vi "UI_visual.vi"() -> ()   [LabVIEW 2017]
uses:
  <vilib>/Analysis/coordinate.llb/Euler Rotation Order.ctl
  <vilib>/Utility/miscctls.llb/LV3DPointTypeDef.ctl
  <vilib>/Analysis/baseanly.llb/Real A x B.vi
  <vilib>/Analysis/Matrix/Numeric/Conversions/Array To Matrix - RA.vi
  <vilib>/Analysis/Matrix/Numeric/Conversions/Array To Matrix - RA2.vi
  <vilib>/Analysis/Matrix/Numeric/Conversions/Matrix To Array - RM.vi
  <vilib>/picture/3D Picture Control/Object/Create Object (drawable).vi
  <vilib>/picture/3D Picture Control/Object/Create Object (name).vi
  <vilib>/picture/3D Picture Control/Object/Add Object (no reference).vi
  <vilib>/picture/3D Picture Control/Helpers/Set Clip Plane (no reference).vi
  <vilib>/picture/3D Picture Control/Helpers/Apply Texture (no reference).vi
  <vilib>/picture/3D Picture Control/NI_3D Picture Control.lvlib
  <vilib>/Analysis/NI_AALPro.lvlib
  <vilib>/Analysis/Matrix/NI_Matrix.lvlib
  <vilib>/Analysis/NI_AALBase.lvlib
panel:
  out "Euler_angles recebidos":dbl[](array[numeric])
  out "Euler Angles":dbl[](array[numeric])
  out "alt":dbl
  out "B-frame":cluster{"X":sgl, "Y":sgl, "Z":sgl}
  out "array":dbl[](array[numeric])
  in  "B-frame Translation 2":cluster{"X":sgl, "Y":sgl, "Z":sgl}
  in  "N-frame rot":dbl[](array[numeric])
  in  "N-frame Translation":cluster{"X":sgl, "Y":sgl, "Z":sgl}
  in  "B-frame Translation":cluster{"X":sgl, "Y":sgl, "Z":sgl}
  in  "Up Direction":T1={"X"=0.0, "Y"=0.0, "Z"=1.0}
  out "3D Picture Control":refnum<vi>(3d-picture)
  in  "error in (no error)":errorcluster
  in  "rotation order":T2 items=["X-Y-Z", "X-Z-Y", "Y-X-Z", "Y-Z-X", "Z-X-Y", "Z-Y-X", "X-Y-X", "X-Z-X", "Y-X-Y", "Y-Z-Y", "Z-X-Z", "Z-Y-Z"]
  in  "Rodar nesta VI":bool
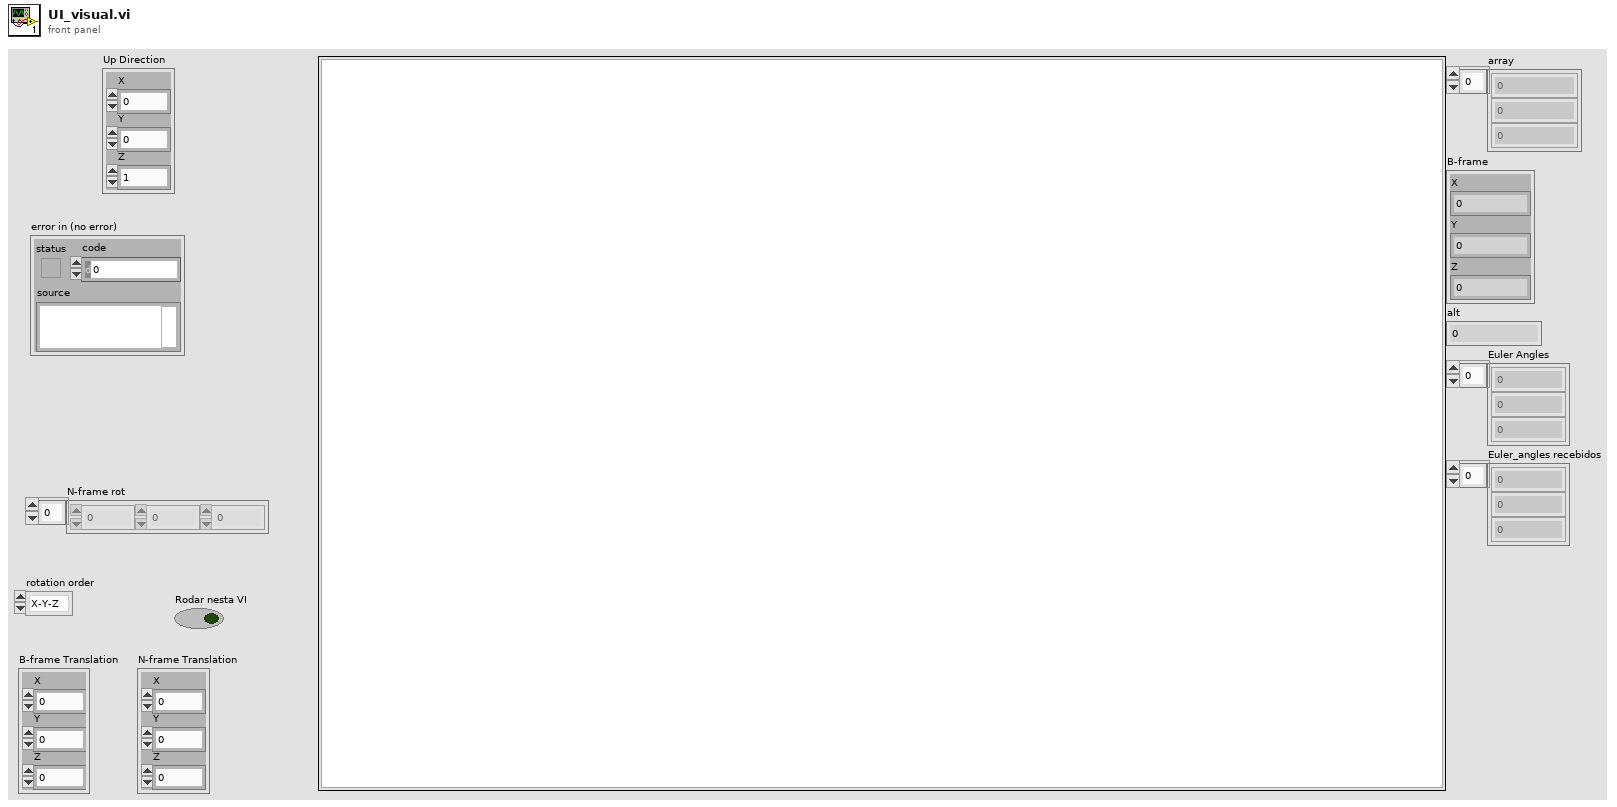
[diagram p1: front panel]
types:
  T1 = typedef "LV3DPointTypeDef.ctl" = cluster{"X":sgl, "Y":sgl, "Z":sgl}
  T2 = typedef "NI_AALPro.lvlib/Euler Rotation Order.ctl" = u16
  T3 = cluster{"Red":sgl, "Green":sgl, "Blue":sgl, "Alpha":sgl}
  T4 = enum16{"As a Decal", "With Modulation", "With Blending", "As a replacement"}
  T5 = enum16{"Inherit Value", "Points", "Wireframe", "Polygons"}
  T6 = typedef "NI_Matrix.lvlib/RealMatrix.ctl" = dbl[][]
  T7 = typedef "imagedata.ctl" = cluster{"image type":i32, "image depth":i32, "image":u8[], "mask":u8[], "colors":u32[], "Rectangle":cluster{"left":i16, "top":i16, "right":i16, "bottom":i16}}
  T8 = cluster{"element":dbl, "element":dbl, "element":dbl}
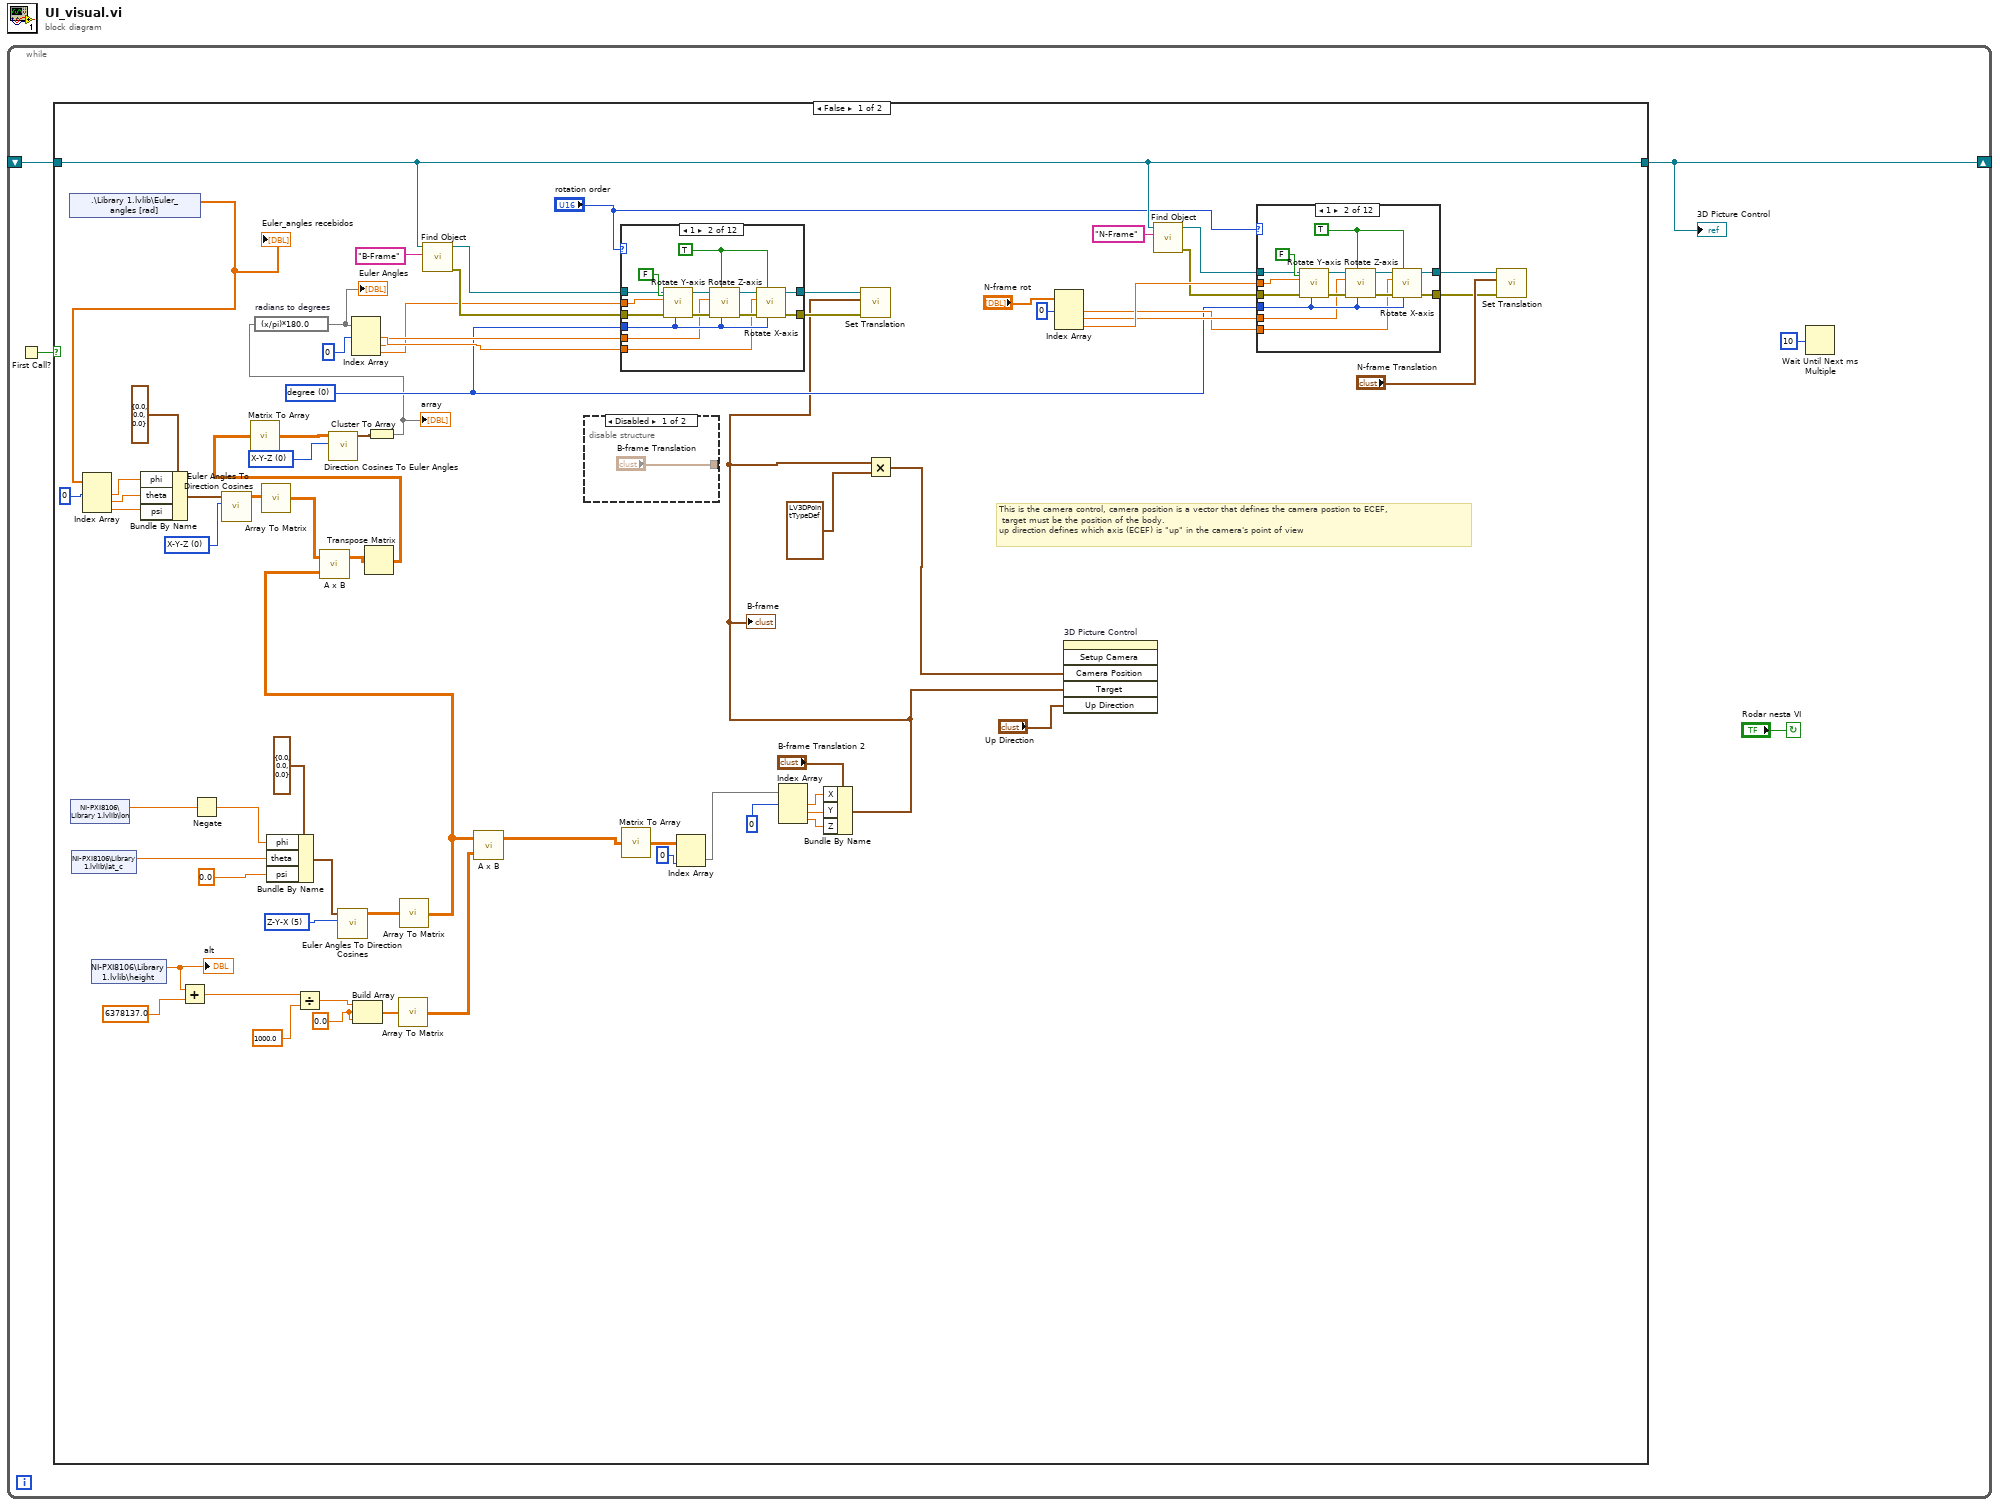
[diagram p0: block diagram]
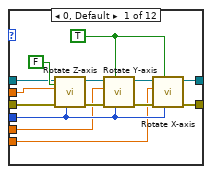
[diagram p3: hidden frame]
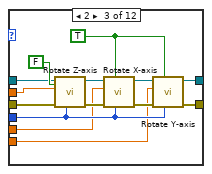
[diagram p4: hidden frame]
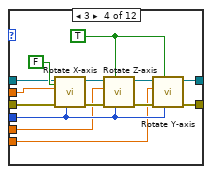
[diagram p5: hidden frame]
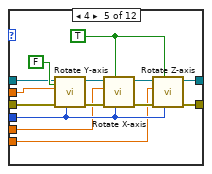
[diagram p6: hidden frame]
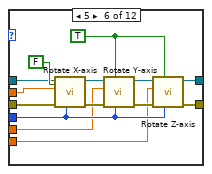
[diagram p7: hidden frame]
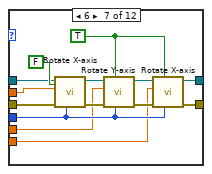
[diagram p8: hidden frame]
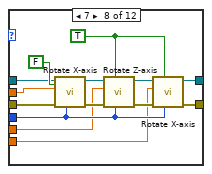
[diagram p9: hidden frame]
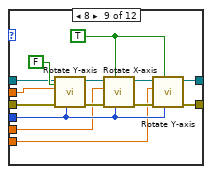
[diagram p10: hidden frame]
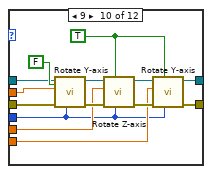
[diagram p11: hidden frame]
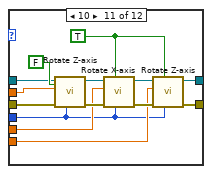
[diagram p12: hidden frame]
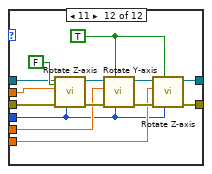
[diagram p13: hidden frame]
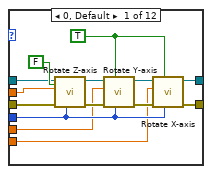
[diagram p14: hidden frame]
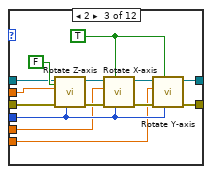
[diagram p15: hidden frame]
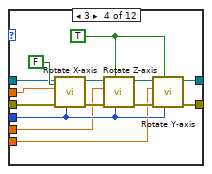
[diagram p16: hidden frame]
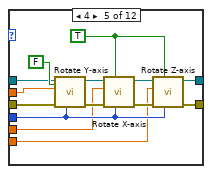
[diagram p17: hidden frame]
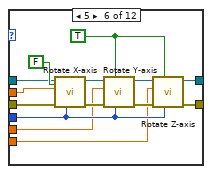
[diagram p18: hidden frame]
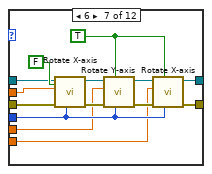
[diagram p19: hidden frame]
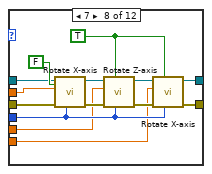
[diagram p20: hidden frame]
diagram:
  n1 = while {
    shift-right: [w2] -> _
    shift-left: _ -> [w3]
    stop <- "Rodar nesta VI" continue-if-true
    n2 = First Call?() -> (First Call?: T/F=w5:bool)
    n3 = case shown="False" w5 {
      tunnel: [w53 w425] -> w2
      tunnel: w3 -> [w53 _]
      frame False {
        w16 = T2 0 items=["X-Y-Z", "X-Z-Y", "Y-X-Z", "Y-Z-X", "Z-X-Y", "Z-Y-X", "X-Y-X", "X-Z-X", "Y-X-Y", "Y-Z-Y", "Z-X-Z", "Z-Y-Z"] ("rotation order")
        w27 = T2 0 items=["X-Y-Z", "X-Z-Y", "Y-X-Z", "Y-Z-X", "Z-X-Y", "Z-Y-X", "X-Y-X", "X-Z-X", "Y-X-Y", "Y-Z-Y", "Z-X-Z", "Z-Y-Z"] ("rotation order")
        w42 = 0.0 ("element")
        w50 = T2 5 items=["X-Y-Z", "X-Z-Y", "Y-X-Z", "Y-Z-X", "Z-X-Y", "Z-Y-X", "X-Y-X", "X-Z-X", "Y-X-Y", "Y-Z-Y", "Z-X-Z", "Z-Y-Z"] ("rotation order")
        w51 = u16 0 items=["degree", "radians"] ("angle unit")
        # "This is the camera control, camera position is a vector that defines the camera postion to ECEF,\n target must be the position of the body. \nup direction defines which axis (ECEF) is \"up\" in the camera's point of view"
        n4 = shared-variable ".\\Library 1.lvlib\\Euler_angles [rad]"() -> (w6:dbl[])  [unwired: 1 in, 1 out]
        "Euler_angles recebidos" <- w6
        n5 = shared-variable "NI-PXI8106\\Library 1.lvlib\\lon"() -> (w10:dbl)  [unwired: 1 in, 1 out]
        n6 = shared-variable "NI-PXI8106\\Library 1.lvlib\\lat_c"() -> (w11:dbl)  [unwired: 1 in, 1 out]
        n7 = Index Array(array=w6, index #1=0 ("index")) -> (element #1=w25:dbl, element #2=w24:dbl, element #3=w23:dbl)  [unwired: 2 in]
        n8 = shared-variable "NI-PXI8106\\Library 1.lvlib\\height"() -> (w46:dbl)  [unwired: 1 in, 1 out]
        "alt" <- w46
        n9 = Bundle By Name(cluster=cluster{"phi":dbl, "theta":dbl, "psi":dbl} {"phi"=0.0, "theta"=0.0, "psi"=0.0} ("Euler Angles"), "phi"=w25, "theta"=w24, "psi"=w23) -> (w28:cluster{"phi":dbl, "theta":dbl, "psi":dbl})
        n10 = Add(x=w46, y=6378137.0) -> (x+y=w44:dbl)
        n11 = Negate(x=w10) -> (-x=w9:dbl)
        n12 = call <vilib>:"Euler Angles To Direction Cosines.vi"("rotation order"=w27, "Euler Angles"=w28) -> ("Direction Cosines"=w22:dbl[][])  [unwired: 8 in, 1 out]
        n13 = call-poly <vilib>:"Array To Matrix.vi"("Real 2D Array"=w22) -> ("Real Matrix"=w21:T6)
        n14 = Bundle By Name(cluster=cluster{"phi":dbl, "theta":dbl, "psi":dbl} {"phi"=0.0, "theta"=0.0, "psi"=0.0} ("Euler Angles"), "phi"=w9, "theta"=w11, "psi"=0.0) -> (w48:cluster{"phi":dbl, "theta":dbl, "psi":dbl})
        n15 = Divide(x=w44, y=1000.0) -> (x/y=w43:dbl)
        n16 = call <vilib>:"Euler Angles To Direction Cosines.vi"("rotation order"=w50, "Euler Angles"=w48) -> ("Direction Cosines"=w39:dbl[][])  [unwired: 8 in, 1 out]
        n17 = Build Array(w43, w42, w42) -> (w41:dbl[])
        n18 = call-poly <vilib>:"Array To Matrix.vi"("Real 1D Array"=w41) -> ("Real Matrix (Column Vector)"=w40:T6)
        n19 = call-poly <vilib>:"Array To Matrix.vi"("Real 2D Array"=w39) -> ("Real Matrix"=w20:T6)
        n20 = call-poly <vilib>:"A x B.vi"("B"=w20, "A"=w21) -> ("A x B"=w19:T6)  [unwired: 1 out]
        n21 = Transpose Matrix(1:w19) -> (0:w18:T6)
        n22 = call-poly <vilib>:"Matrix To Array.vi"("Real Matrix"=w18) -> ("Real 2D Array"=w17:dbl[][])
        n23 = call <vilib>:"Direction Cosines To Euler Angles.vi"("rotation order"=w16, "Direction Cosines"=w17) -> ("Euler Angles"=w15:cluster{"phi":dbl, "theta":dbl, "psi":dbl})  [unwired: 8 in, 1 out]
        n24 = Cluster To Array(cluster=w15) -> (array=w13:dbl[])
        "array" <- w13
        n25 = expression code="(x/pi)*180.0" "radians to degrees"(w13) -> (w14:dbl[])
        "Euler Angles" <- w14
        n26 = Index Array(array=w14, index #1=0 ("index")) -> (element #1=w74:dbl, element #2=w71:dbl, element #3=w70:dbl)  [unwired: 2 in]
        n27 = call <vilib>:"Find Object.vi"("Object Name"="B-Frame", "Scene Refnum"=w53) -> ("error out"=w72:errorcluster, "Object Refnum"=w73:refnum<vi>)  [unwired: 8 in]
        n28 = call-poly <vilib>:"A x B.vi"("B"=w40, "A"=w20) -> ("A x B"=w36:T6)  [unwired: 1 out]
        n29 = disable-structure shown="Disabled" {
          disable-tunnel: ["B-frame Translation" _] -> _
          frame Disabled {
          }
          frame Enabled {
          }
        }
        n30 = case shown="1" "rotation order" {
          tunnel: w74 -> [w249 w265 w279 w293 w303 w321 w335 w349 w363 w374 w388 w402]
          tunnel: w73 -> [w252 w262 w275 w289 w307 w317 w334 w348 w359 w378 w392 w406]
          tunnel: w72 -> [w251 w261 w276 w290 w306 w318 w333 w347 w360 w377 w391 w405]
          tunnel: w71 -> [w248 w263 w278 w292 w304 w320 w331 w345 w362 w375 w389 w404]
          tunnel: w70 -> [w247 w264 w277 w291 w305 w319 w332 w346 w361 w376 w390 w403]
          tunnel: w51 -> [w250 w266 w280 w294 w308 w322 w336 w350 w364 w373 w387 w401]
          tunnel: [w246 w260 w274 w288 w302 w316 w330 w344 w358 w372 w386 w400] -> w68
          tunnel: [w245 w259 w273 w287 w301 w315 w329 w343 w357 w371 w385 w399] -> w67
          frame 0, Default {
            w258 = TRUE ("Relative?")
            n31 = call <vilib>:"Rotate Z-axis.vi"("angle unit"=w250, "Relative?"=FALSE, "error in (no error)"=w251, "angle"=w247, "Scene Object In"=w252) -> ("error out"=w255:errorcluster, "Scene Object Out"=w256:refnum<vi>)  [unwired: 5 in]
            n32 = call <vilib>:"Rotate Y-axis.vi"("angle unit"=w250, "Relative?"=w258, "error in (no error)"=w255, "angle"=w248, "Scene Object In"=w256) -> ("error out"=w254:errorcluster, "Scene Object Out"=w253:refnum<vi>)  [unwired: 5 in]
            n33 = call <vilib>:"Rotate X-axis.vi"("angle unit"=w250, "Relative?"=w258, "error in (no error)"=w254, "angle"=w249, "Scene Object In"=w253) -> ("error out"=w245:errorcluster, "Scene Object Out"=w246:refnum<vi>)  [unwired: 5 in]
          }
          frame 1 {
            w269 = TRUE ("Relative?")
            n34 = call <vilib>:"Rotate Y-axis.vi"("angle unit"=w266, "Relative?"=FALSE, "error in (no error)"=w261, "angle"=w264, "Scene Object In"=w262) -> ("error out"=w270:errorcluster, "Scene Object Out"=w271:refnum<vi>)  [unwired: 5 in]
            n35 = call <vilib>:"Rotate Z-axis.vi"("angle unit"=w266, "Relative?"=w269, "error in (no error)"=w270, "angle"=w263, "Scene Object In"=w271) -> ("error out"=w267:errorcluster, "Scene Object Out"=w268:refnum<vi>)  [unwired: 5 in]
            n36 = call <vilib>:"Rotate X-axis.vi"("angle unit"=w266, "Relative?"=w269, "error in (no error)"=w267, "angle"=w265, "Scene Object In"=w268) -> ("error out"=w259:errorcluster, "Scene Object Out"=w260:refnum<vi>)  [unwired: 5 in]
          }
          frame 2 {
            w281 = TRUE ("Relative?")
            n37 = call <vilib>:"Rotate Z-axis.vi"("angle unit"=w280, "Relative?"=FALSE, "error in (no error)"=w276, "angle"=w277, "Scene Object In"=w275) -> ("error out"=w284:errorcluster, "Scene Object Out"=w285:refnum<vi>)  [unwired: 5 in]
            n38 = call <vilib>:"Rotate X-axis.vi"("angle unit"=w280, "Relative?"=w281, "error in (no error)"=w284, "angle"=w278, "Scene Object In"=w285) -> ("error out"=w282:errorcluster, "Scene Object Out"=w283:refnum<vi>)  [unwired: 5 in]
            n39 = call <vilib>:"Rotate Y-axis.vi"("angle unit"=w280, "Relative?"=w281, "error in (no error)"=w282, "angle"=w279, "Scene Object In"=w283) -> ("error out"=w273:errorcluster, "Scene Object Out"=w274:refnum<vi>)  [unwired: 5 in]
          }
          frame 3 {
            w299 = TRUE ("Relative?")
            n40 = call <vilib>:"Rotate X-axis.vi"("angle unit"=w294, "Relative?"=FALSE, "error in (no error)"=w290, "angle"=w291, "Scene Object In"=w289) -> ("error out"=w297:errorcluster, "Scene Object Out"=w298:refnum<vi>)  [unwired: 5 in]
            n41 = call <vilib>:"Rotate Z-axis.vi"("angle unit"=w294, "Relative?"=w299, "error in (no error)"=w297, "angle"=w292, "Scene Object In"=w298) -> ("error out"=w295:errorcluster, "Scene Object Out"=w296:refnum<vi>)  [unwired: 5 in]
            n42 = call <vilib>:"Rotate Y-axis.vi"("angle unit"=w294, "Relative?"=w299, "error in (no error)"=w295, "angle"=w293, "Scene Object In"=w296) -> ("error out"=w287:errorcluster, "Scene Object Out"=w288:refnum<vi>)  [unwired: 5 in]
          }
          frame 4 {
            w313 = TRUE ("Relative?")
            n43 = call <vilib>:"Rotate Y-axis.vi"("angle unit"=w308, "Relative?"=FALSE, "error in (no error)"=w306, "angle"=w305, "Scene Object In"=w307) -> ("error out"=w309:errorcluster, "Scene Object Out"=w310:refnum<vi>)  [unwired: 5 in]
            n44 = call <vilib>:"Rotate X-axis.vi"("angle unit"=w308, "Relative?"=w313, "error in (no error)"=w309, "angle"=w304, "Scene Object In"=w310) -> ("error out"=w312:errorcluster, "Scene Object Out"=w311:refnum<vi>)  [unwired: 5 in]
            n45 = call <vilib>:"Rotate Z-axis.vi"("angle unit"=w308, "Relative?"=w313, "error in (no error)"=w312, "angle"=w303, "Scene Object In"=w311) -> ("error out"=w301:errorcluster, "Scene Object Out"=w302:refnum<vi>)  [unwired: 5 in]
          }
          frame 5 {
            w326 = TRUE ("Relative?")
            n46 = call <vilib>:"Rotate X-axis.vi"("angle unit"=w322, "Relative?"=FALSE, "error in (no error)"=w318, "angle"=w319, "Scene Object In"=w317) -> ("error out"=w324:errorcluster, "Scene Object Out"=w325:refnum<vi>)  [unwired: 5 in]
            n47 = call <vilib>:"Rotate Y-axis.vi"("angle unit"=w322, "Relative?"=w326, "error in (no error)"=w324, "angle"=w320, "Scene Object In"=w325) -> ("error out"=w328:errorcluster, "Scene Object Out"=w327:refnum<vi>)  [unwired: 5 in]
            n48 = call <vilib>:"Rotate Z-axis.vi"("angle unit"=w322, "Relative?"=w326, "error in (no error)"=w328, "angle"=w321, "Scene Object In"=w327) -> ("error out"=w315:errorcluster, "Scene Object Out"=w316:refnum<vi>)  [unwired: 5 in]
          }
          frame 6 {
            w339 = TRUE ("Relative?")
            n49 = call <vilib>:"Rotate X-axis.vi"("angle unit"=w336, "Relative?"=FALSE, "error in (no error)"=w333, "angle"=w332, "Scene Object In"=w334) -> ("error out"=w341:errorcluster, "Scene Object Out"=w342:refnum<vi>)  [unwired: 5 in]
            n50 = call <vilib>:"Rotate Y-axis.vi"("angle unit"=w336, "Relative?"=w339, "error in (no error)"=w341, "angle"=w331, "Scene Object In"=w342) -> ("error out"=w337:errorcluster, "Scene Object Out"=w338:refnum<vi>)  [unwired: 5 in]
            n51 = call <vilib>:"Rotate X-axis.vi"("angle unit"=w336, "Relative?"=w339, "error in (no error)"=w337, "angle"=w335, "Scene Object In"=w338) -> ("error out"=w329:errorcluster, "Scene Object Out"=w330:refnum<vi>)  [unwired: 5 in]
          }
          frame 7 {
            w355 = TRUE ("Relative?")
            n52 = call <vilib>:"Rotate X-axis.vi"("angle unit"=w350, "Relative?"=FALSE, "error in (no error)"=w347, "angle"=w346, "Scene Object In"=w348) -> ("error out"=w353:errorcluster, "Scene Object Out"=w354:refnum<vi>)  [unwired: 5 in]
            n53 = call <vilib>:"Rotate Z-axis.vi"("angle unit"=w350, "Relative?"=w355, "error in (no error)"=w353, "angle"=w345, "Scene Object In"=w354) -> ("error out"=w352:errorcluster, "Scene Object Out"=w351:refnum<vi>)  [unwired: 5 in]
            n54 = call <vilib>:"Rotate X-axis.vi"("angle unit"=w350, "Relative?"=w355, "error in (no error)"=w352, "angle"=w349, "Scene Object In"=w351) -> ("error out"=w343:errorcluster, "Scene Object Out"=w344:refnum<vi>)  [unwired: 5 in]
          }
          frame 8 {
            w369 = TRUE ("Relative?")
            n55 = call <vilib>:"Rotate Y-axis.vi"("angle unit"=w364, "Relative?"=FALSE, "error in (no error)"=w360, "angle"=w361, "Scene Object In"=w359) -> ("error out"=w367:errorcluster, "Scene Object Out"=w368:refnum<vi>)  [unwired: 5 in]
            n56 = call <vilib>:"Rotate X-axis.vi"("angle unit"=w364, "Relative?"=w369, "error in (no error)"=w367, "angle"=w362, "Scene Object In"=w368) -> ("error out"=w366:errorcluster, "Scene Object Out"=w365:refnum<vi>)  [unwired: 5 in]
            n57 = call <vilib>:"Rotate Y-axis.vi"("angle unit"=w364, "Relative?"=w369, "error in (no error)"=w366, "angle"=w363, "Scene Object In"=w365) -> ("error out"=w357:errorcluster, "Scene Object Out"=w358:refnum<vi>)  [unwired: 5 in]
          }
          frame 9 {
            w383 = TRUE ("Relative?")
            n58 = call <vilib>:"Rotate Y-axis.vi"("angle unit"=w373, "Relative?"=FALSE, "error in (no error)"=w377, "angle"=w376, "Scene Object In"=w378) -> ("error out"=w381:errorcluster, "Scene Object Out"=w382:refnum<vi>)  [unwired: 5 in]
            n59 = call <vilib>:"Rotate Z-axis.vi"("angle unit"=w373, "Relative?"=w383, "error in (no error)"=w381, "angle"=w375, "Scene Object In"=w382) -> ("error out"=w380:errorcluster, "Scene Object Out"=w379:refnum<vi>)  [unwired: 5 in]
            n60 = call <vilib>:"Rotate Y-axis.vi"("angle unit"=w373, "Relative?"=w383, "error in (no error)"=w380, "angle"=w374, "Scene Object In"=w379) -> ("error out"=w371:errorcluster, "Scene Object Out"=w372:refnum<vi>)  [unwired: 5 in]
          }
          frame 10 {
            w397 = TRUE ("Relative?")
            n61 = call <vilib>:"Rotate Z-axis.vi"("angle unit"=w387, "Relative?"=FALSE, "error in (no error)"=w391, "angle"=w390, "Scene Object In"=w392) -> ("error out"=w395:errorcluster, "Scene Object Out"=w396:refnum<vi>)  [unwired: 5 in]
            n62 = call <vilib>:"Rotate X-axis.vi"("angle unit"=w387, "Relative?"=w397, "error in (no error)"=w395, "angle"=w389, "Scene Object In"=w396) -> ("error out"=w394:errorcluster, "Scene Object Out"=w393:refnum<vi>)  [unwired: 5 in]
            n63 = call <vilib>:"Rotate Z-axis.vi"("angle unit"=w387, "Relative?"=w397, "error in (no error)"=w394, "angle"=w388, "Scene Object In"=w393) -> ("error out"=w385:errorcluster, "Scene Object Out"=w386:refnum<vi>)  [unwired: 5 in]
          }
          frame 11 {
            w411 = TRUE ("Relative?")
            n64 = call <vilib>:"Rotate Z-axis.vi"("angle unit"=w401, "Relative?"=FALSE, "error in (no error)"=w405, "angle"=w403, "Scene Object In"=w406) -> ("error out"=w409:errorcluster, "Scene Object Out"=w410:refnum<vi>)  [unwired: 5 in]
            n65 = call <vilib>:"Rotate Y-axis.vi"("angle unit"=w401, "Relative?"=w411, "error in (no error)"=w409, "angle"=w404, "Scene Object In"=w410) -> ("error out"=w408:errorcluster, "Scene Object Out"=w407:refnum<vi>)  [unwired: 5 in]
            n66 = call <vilib>:"Rotate Z-axis.vi"("angle unit"=w401, "Relative?"=w411, "error in (no error)"=w408, "angle"=w402, "Scene Object In"=w407) -> ("error out"=w399:errorcluster, "Scene Object Out"=w400:refnum<vi>)  [unwired: 5 in]
          }
        }
        n67 = call-poly <vilib>:"Matrix To Array.vi"("Real Matrix"=w36) -> ("Real 2D Array"=w38:dbl[][])
        n68 = Index Array(array=w38, index (col)=0 ("index (row)")) -> (element=w35:dbl[])  [unwired: 1 in]
        n69 = Index Array(array=w35, index #1=0 ("index")) -> (element #1=w32:dbl, element #2=w31:dbl, element #3=w30:dbl)  [unwired: 2 in]
        n70 = Bundle By Name(cluster="B-frame Translation 2", "X"=w32, "Y"=w31, "Z"=w30) -> (w7:cluster{"X":sgl, "Y":sgl, "Z":sgl})
        "B-frame" <- w7
        n71 = call <vilib>:"Set Translation.vi"("error in (no error)"=w67, "Translation"=w7, "Scene Object"=w68) -> ()  [unwired: 7 in, 2 out]
        n72 = Multiply(x=w7, y=T1 {"X"=1.001, "Y"=1.001, "Z"=1.001} ("Camera Position")) -> (x*y=w65:T1)
        n73 = Index Array(array="N-frame rot", index #1=0 ("index")) -> (element #1=w56:dbl, element #2=w59:dbl, element #3=w60:dbl)  [unwired: 2 in]
        n74 = invoke on="3D Picture Control" class="SceneGraphDisp (strict)" method="Setup Camera"("Camera Position"=w65, "Target"=w7, "Up Direction"="Up Direction") -> ()  [unwired: 3 in, 6 out]
        n75 = call <vilib>:"Find Object.vi"("Object Name"="N-Frame", "Scene Refnum"=w53) -> ("error out"=w58:errorcluster, "Object Refnum"=w57:refnum<vi>)  [unwired: 8 in]
        n76 = case shown="1" "rotation order" {
          tunnel: w56 -> [w81 w97 w111 w125 w135 w153 w167 w181 w195 w206 w220 w234]
          tunnel: w57 -> [w84 w94 w107 w121 w139 w149 w166 w180 w191 w210 w224 w238]
          tunnel: w58 -> [w83 w93 w108 w122 w138 w150 w165 w179 w192 w209 w223 w237]
          tunnel: w59 -> [w80 w95 w110 w124 w136 w152 w163 w177 w194 w207 w221 w236]
          tunnel: w60 -> [w79 w96 w109 w123 w137 w151 w164 w178 w193 w208 w222 w235]
          tunnel: w51 -> [w82 w98 w112 w126 w140 w154 w168 w182 w196 w205 w219 w233]
          tunnel: [w78 w92 w106 w120 w134 w148 w162 w176 w190 w204 w218 w232] -> w62
          tunnel: [w77 w91 w105 w119 w133 w147 w161 w175 w189 w203 w217 w231] -> w63
          frame 0, Default {
            w90 = TRUE ("Relative?")
            n77 = call <vilib>:"Rotate Z-axis.vi"("angle unit"=w82, "Relative?"=FALSE, "error in (no error)"=w83, "angle"=w79, "Scene Object In"=w84) -> ("error out"=w87:errorcluster, "Scene Object Out"=w88:refnum<vi>)  [unwired: 5 in]
            n78 = call <vilib>:"Rotate Y-axis.vi"("angle unit"=w82, "Relative?"=w90, "error in (no error)"=w87, "angle"=w80, "Scene Object In"=w88) -> ("error out"=w86:errorcluster, "Scene Object Out"=w85:refnum<vi>)  [unwired: 5 in]
            n79 = call <vilib>:"Rotate X-axis.vi"("angle unit"=w82, "Relative?"=w90, "error in (no error)"=w86, "angle"=w81, "Scene Object In"=w85) -> ("error out"=w77:errorcluster, "Scene Object Out"=w78:refnum<vi>)  [unwired: 5 in]
          }
          frame 1 {
            w101 = TRUE ("Relative?")
            n80 = call <vilib>:"Rotate Y-axis.vi"("angle unit"=w98, "Relative?"=FALSE, "error in (no error)"=w93, "angle"=w96, "Scene Object In"=w94) -> ("error out"=w102:errorcluster, "Scene Object Out"=w103:refnum<vi>)  [unwired: 5 in]
            n81 = call <vilib>:"Rotate Z-axis.vi"("angle unit"=w98, "Relative?"=w101, "error in (no error)"=w102, "angle"=w95, "Scene Object In"=w103) -> ("error out"=w99:errorcluster, "Scene Object Out"=w100:refnum<vi>)  [unwired: 5 in]
            n82 = call <vilib>:"Rotate X-axis.vi"("angle unit"=w98, "Relative?"=w101, "error in (no error)"=w99, "angle"=w97, "Scene Object In"=w100) -> ("error out"=w91:errorcluster, "Scene Object Out"=w92:refnum<vi>)  [unwired: 5 in]
          }
          frame 2 {
            w113 = TRUE ("Relative?")
            n83 = call <vilib>:"Rotate Z-axis.vi"("angle unit"=w112, "Relative?"=FALSE, "error in (no error)"=w108, "angle"=w109, "Scene Object In"=w107) -> ("error out"=w116:errorcluster, "Scene Object Out"=w117:refnum<vi>)  [unwired: 5 in]
            n84 = call <vilib>:"Rotate X-axis.vi"("angle unit"=w112, "Relative?"=w113, "error in (no error)"=w116, "angle"=w110, "Scene Object In"=w117) -> ("error out"=w114:errorcluster, "Scene Object Out"=w115:refnum<vi>)  [unwired: 5 in]
            n85 = call <vilib>:"Rotate Y-axis.vi"("angle unit"=w112, "Relative?"=w113, "error in (no error)"=w114, "angle"=w111, "Scene Object In"=w115) -> ("error out"=w105:errorcluster, "Scene Object Out"=w106:refnum<vi>)  [unwired: 5 in]
          }
          frame 3 {
            w131 = TRUE ("Relative?")
            n86 = call <vilib>:"Rotate X-axis.vi"("angle unit"=w126, "Relative?"=FALSE, "error in (no error)"=w122, "angle"=w123, "Scene Object In"=w121) -> ("error out"=w129:errorcluster, "Scene Object Out"=w130:refnum<vi>)  [unwired: 5 in]
            n87 = call <vilib>:"Rotate Z-axis.vi"("angle unit"=w126, "Relative?"=w131, "error in (no error)"=w129, "angle"=w124, "Scene Object In"=w130) -> ("error out"=w127:errorcluster, "Scene Object Out"=w128:refnum<vi>)  [unwired: 5 in]
            n88 = call <vilib>:"Rotate Y-axis.vi"("angle unit"=w126, "Relative?"=w131, "error in (no error)"=w127, "angle"=w125, "Scene Object In"=w128) -> ("error out"=w119:errorcluster, "Scene Object Out"=w120:refnum<vi>)  [unwired: 5 in]
          }
          frame 4 {
            w145 = TRUE ("Relative?")
            n89 = call <vilib>:"Rotate Y-axis.vi"("angle unit"=w140, "Relative?"=FALSE, "error in (no error)"=w138, "angle"=w137, "Scene Object In"=w139) -> ("error out"=w141:errorcluster, "Scene Object Out"=w142:refnum<vi>)  [unwired: 5 in]
            n90 = call <vilib>:"Rotate X-axis.vi"("angle unit"=w140, "Relative?"=w145, "error in (no error)"=w141, "angle"=w136, "Scene Object In"=w142) -> ("error out"=w144:errorcluster, "Scene Object Out"=w143:refnum<vi>)  [unwired: 5 in]
            n91 = call <vilib>:"Rotate Z-axis.vi"("angle unit"=w140, "Relative?"=w145, "error in (no error)"=w144, "angle"=w135, "Scene Object In"=w143) -> ("error out"=w133:errorcluster, "Scene Object Out"=w134:refnum<vi>)  [unwired: 5 in]
          }
          frame 5 {
            w158 = TRUE ("Relative?")
            n92 = call <vilib>:"Rotate X-axis.vi"("angle unit"=w154, "Relative?"=FALSE, "error in (no error)"=w150, "angle"=w151, "Scene Object In"=w149) -> ("error out"=w156:errorcluster, "Scene Object Out"=w157:refnum<vi>)  [unwired: 5 in]
            n93 = call <vilib>:"Rotate Y-axis.vi"("angle unit"=w154, "Relative?"=w158, "error in (no error)"=w156, "angle"=w152, "Scene Object In"=w157) -> ("error out"=w160:errorcluster, "Scene Object Out"=w159:refnum<vi>)  [unwired: 5 in]
            n94 = call <vilib>:"Rotate Z-axis.vi"("angle unit"=w154, "Relative?"=w158, "error in (no error)"=w160, "angle"=w153, "Scene Object In"=w159) -> ("error out"=w147:errorcluster, "Scene Object Out"=w148:refnum<vi>)  [unwired: 5 in]
          }
          frame 6 {
            w171 = TRUE ("Relative?")
            n95 = call <vilib>:"Rotate X-axis.vi"("angle unit"=w168, "Relative?"=FALSE, "error in (no error)"=w165, "angle"=w164, "Scene Object In"=w166) -> ("error out"=w173:errorcluster, "Scene Object Out"=w174:refnum<vi>)  [unwired: 5 in]
            n96 = call <vilib>:"Rotate Y-axis.vi"("angle unit"=w168, "Relative?"=w171, "error in (no error)"=w173, "angle"=w163, "Scene Object In"=w174) -> ("error out"=w169:errorcluster, "Scene Object Out"=w170:refnum<vi>)  [unwired: 5 in]
            n97 = call <vilib>:"Rotate X-axis.vi"("angle unit"=w168, "Relative?"=w171, "error in (no error)"=w169, "angle"=w167, "Scene Object In"=w170) -> ("error out"=w161:errorcluster, "Scene Object Out"=w162:refnum<vi>)  [unwired: 5 in]
          }
          frame 7 {
            w187 = TRUE ("Relative?")
            n98 = call <vilib>:"Rotate X-axis.vi"("angle unit"=w182, "Relative?"=FALSE, "error in (no error)"=w179, "angle"=w178, "Scene Object In"=w180) -> ("error out"=w185:errorcluster, "Scene Object Out"=w186:refnum<vi>)  [unwired: 5 in]
            n99 = call <vilib>:"Rotate Z-axis.vi"("angle unit"=w182, "Relative?"=w187, "error in (no error)"=w185, "angle"=w177, "Scene Object In"=w186) -> ("error out"=w184:errorcluster, "Scene Object Out"=w183:refnum<vi>)  [unwired: 5 in]
            n100 = call <vilib>:"Rotate X-axis.vi"("angle unit"=w182, "Relative?"=w187, "error in (no error)"=w184, "angle"=w181, "Scene Object In"=w183) -> ("error out"=w175:errorcluster, "Scene Object Out"=w176:refnum<vi>)  [unwired: 5 in]
          }
          frame 8 {
            w201 = TRUE ("Relative?")
            n101 = call <vilib>:"Rotate Y-axis.vi"("angle unit"=w196, "Relative?"=FALSE, "error in (no error)"=w192, "angle"=w193, "Scene Object In"=w191) -> ("error out"=w199:errorcluster, "Scene Object Out"=w200:refnum<vi>)  [unwired: 5 in]
            n102 = call <vilib>:"Rotate X-axis.vi"("angle unit"=w196, "Relative?"=w201, "error in (no error)"=w199, "angle"=w194, "Scene Object In"=w200) -> ("error out"=w198:errorcluster, "Scene Object Out"=w197:refnum<vi>)  [unwired: 5 in]
            n103 = call <vilib>:"Rotate Y-axis.vi"("angle unit"=w196, "Relative?"=w201, "error in (no error)"=w198, "angle"=w195, "Scene Object In"=w197) -> ("error out"=w189:errorcluster, "Scene Object Out"=w190:refnum<vi>)  [unwired: 5 in]
          }
          frame 9 {
            w215 = TRUE ("Relative?")
            n104 = call <vilib>:"Rotate Y-axis.vi"("angle unit"=w205, "Relative?"=FALSE, "error in (no error)"=w209, "angle"=w208, "Scene Object In"=w210) -> ("error out"=w213:errorcluster, "Scene Object Out"=w214:refnum<vi>)  [unwired: 5 in]
            n105 = call <vilib>:"Rotate Z-axis.vi"("angle unit"=w205, "Relative?"=w215, "error in (no error)"=w213, "angle"=w207, "Scene Object In"=w214) -> ("error out"=w212:errorcluster, "Scene Object Out"=w211:refnum<vi>)  [unwired: 5 in]
            n106 = call <vilib>:"Rotate Y-axis.vi"("angle unit"=w205, "Relative?"=w215, "error in (no error)"=w212, "angle"=w206, "Scene Object In"=w211) -> ("error out"=w203:errorcluster, "Scene Object Out"=w204:refnum<vi>)  [unwired: 5 in]
          }
          frame 10 {
            w229 = TRUE ("Relative?")
            n107 = call <vilib>:"Rotate Z-axis.vi"("angle unit"=w219, "Relative?"=FALSE, "error in (no error)"=w223, "angle"=w222, "Scene Object In"=w224) -> ("error out"=w227:errorcluster, "Scene Object Out"=w228:refnum<vi>)  [unwired: 5 in]
            n108 = call <vilib>:"Rotate X-axis.vi"("angle unit"=w219, "Relative?"=w229, "error in (no error)"=w227, "angle"=w221, "Scene Object In"=w228) -> ("error out"=w226:errorcluster, "Scene Object Out"=w225:refnum<vi>)  [unwired: 5 in]
            n109 = call <vilib>:"Rotate Z-axis.vi"("angle unit"=w219, "Relative?"=w229, "error in (no error)"=w226, "angle"=w220, "Scene Object In"=w225) -> ("error out"=w217:errorcluster, "Scene Object Out"=w218:refnum<vi>)  [unwired: 5 in]
          }
          frame 11 {
            w243 = TRUE ("Relative?")
            n110 = call <vilib>:"Rotate Z-axis.vi"("angle unit"=w233, "Relative?"=FALSE, "error in (no error)"=w237, "angle"=w235, "Scene Object In"=w238) -> ("error out"=w241:errorcluster, "Scene Object Out"=w242:refnum<vi>)  [unwired: 5 in]
            n111 = call <vilib>:"Rotate Y-axis.vi"("angle unit"=w233, "Relative?"=w243, "error in (no error)"=w241, "angle"=w236, "Scene Object In"=w242) -> ("error out"=w240:errorcluster, "Scene Object Out"=w239:refnum<vi>)  [unwired: 5 in]
            n112 = call <vilib>:"Rotate Z-axis.vi"("angle unit"=w233, "Relative?"=w243, "error in (no error)"=w240, "angle"=w234, "Scene Object In"=w239) -> ("error out"=w231:errorcluster, "Scene Object Out"=w232:refnum<vi>)  [unwired: 5 in]
          }
        }
        n113 = call <vilib>:"Set Translation.vi"("error in (no error)"=w63, "Translation"="N-frame Translation", "Scene Object"=w62) -> ()  [unwired: 7 in, 2 out]
      }
      frame True {
        w475 = sgl 0.0 ("A")
        w497 = 10 ("dimension size")
        w503 = sgl 1.0 ("Row Interval")
        # "Branco"
        # "Cria o frame do corpo"
        # "Cria o frame de navegação"
        # "Underneath Clipping\nPlane: z = 0"
        # "This loads the texture map and\nreadies it to use on the ground."
        # "Use the random height matrix\nto generate a height grid."
        n114 = Current VI's Path() -> (path=w498:path)
        n115 = Initialize Array(0.0 ("element"), w497, w497) -> (w495:dbl[][])
        n116 = Strip Path(path=w498) -> (stripped path=w499:path)  [unwired: 1 out]
        n117 = Build Path(base path=w499, name or relative path="floor2.png") -> (appended path=w501:path)
        n118 = call <vilib>:"Create Height Field.vi"("Column Interval"=w503, "Row Interval"=w503, "Data"=w495) -> ("error out"=w480:errorcluster, "New Height Field Refnum"=w490:refnum<vi>)  [unwired: 1 in, 6 out]
        n119 = call <vilib>:"Read PNG File.vi"("path to PNG file"=w501) -> ("error out"=w482:errorcluster, "image data"=w491:T7)  [unwired: 1 in, 8 out]
        n120 = call-poly <vilib>:"Create Object.vi"("error in (no error)"=w480, "Geometry"=w490, "Name"="Base") -> ("error out"=w481:errorcluster, "Scene:New Object"=w492:refnum<vi>)  [unwired: 7 in]
        n121 = Current VI's Path() -> (path=w422:path)
        n122 = disable-structure shown="Enabled" {
          disable-tunnel: [w512 w514] -> w494
          disable-tunnel: w492 -> [w511 w514]
          disable-tunnel: w491 -> [w510 _]
          disable-tunnel: [w509 w513] -> w483
          disable-tunnel: w482 -> [w508 _]
          disable-tunnel: w481 -> [w507 w513]
          frame Disabled {
            n123 = Merge Errors(w507, w508) -> (w504:errorcluster)
            n124 = call-poly <vilib>:"Apply Texture.vi"("Horizontal Wrap Mode"=enum16{"Clamp", "Repeat"}."Repeat", "error in (no error)"=w504, "Apply Mode"=T4."As a Decal", "Image Data"=w510, "Scene Object In"=w511) -> ("error out"=w509:errorcluster, "Scene Object Out"=w512:refnum<vi>)  [unwired: 5 in]
          }
          frame Enabled {
          }
        }
        n125 = Strip Path(path=w422) -> (stripped path=w421:path)  [unwired: 1 out]
        n126 = Build Path(base path=w421, name or relative path="world32k2.bmp") -> (appended path=w419:path)
        n127 = Bundle("element"=0.0, "element"=0.0, "element"=0.0) -> (w502:T8)  [unwired: 1 out]
        n128 = call <vilib>:"Create 3D Axis.vi"("Axis label?"=TRUE, "Color"=T3 {"Red"=0.0, "Green"=1.0, "Blue"=0.0, "Alpha"=1.0}, "Length"=sgl 1.0 ("Radius"), "Name"="B-Frame") -> ("error out"=w453:errorcluster, "New Object Refnum"=w454:refnum<vi>)  [unwired: 6 in]
        n129 = call <vilib>:"Create 3D Axis.vi"("Axis label?"=TRUE, "Color"=T3 {"Red"=1.0, "Green"=1.0, "Blue"=1.0, "Alpha"=1.0}, "Length"=sgl 1.0 ("Radius"), "Name"="N-Frame") -> ("error out"=w430:errorcluster, "New Object Refnum"=w429:refnum<vi>)  [unwired: 6 in]
        n130 = call <vilib>:"Set Translation.vi"("error in (no error)"=w483, "Translation"=w502, "Scene Object"=w494) -> ("error out"=w484:errorcluster, "Translated Object"=w488:refnum<vi>)  [unwired: 7 out]
        n131 = call-poly <vilib>:"Create Object.vi"("error in (no error)"="error in (no error)", "Name"="world") -> ("error out"=w486:errorcluster, "Scene:New Object"=w487:refnum<vi>)  [unwired: 8 in]
        n132 = call-poly <vilib>:"Create Object.vi"("Name"="Corpo") -> ("error out"=w440:errorcluster, "Scene:New Object"=w439:refnum<vi>)  [unwired: 9 in]
        n133 = call-poly <vilib>:"Create Object.vi"("Name"="sky") -> ("error out"=w416:errorcluster, "Scene:New Object"=w417:refnum<vi>)  [unwired: 9 in]
        n134 = Merge Errors(w486, w484) -> (w485:errorcluster)
        n135 = call <vilib>:"Read BMP File.vi"("path to BMP file"=w419) -> ("image data"=w418:T7)  [unwired: 8 in, 2 out]
        n136 = disable-structure shown="Enabled" {
          disable-tunnel: w440 -> [w542 w549]
          disable-tunnel: w439 -> [w541 w550]
          disable-tunnel: [w540 w550] -> w436
          disable-tunnel: [w539 w549] -> w435
          frame Disabled {
            w545 = -90.0 ("angle")
            w546 = u16 0 items=["degree", "radians"] ("angle unit")
            n137 = call <vilib>:"Rotate Y-axis.vi"("angle unit"=w546, "Relative?"=FALSE, "error in (no error)"=w542, "angle"=w545, "Scene Object In"=w541) -> ("error out"=w548:errorcluster, "Scene Object Out"=w547:refnum<vi>)  [unwired: 5 in]
            n138 = call <vilib>:"Rotate Z-axis.vi"("angle unit"=w546, "Relative?"=TRUE, "error in (no error)"=w548, "angle"=w545, "Scene Object In"=w547) -> ("error out"=w539:errorcluster, "Scene Object Out"=w540:refnum<vi>)  [unwired: 5 in]
          }
          frame Enabled {
          }
        }
        n139 = disable-structure shown="Enabled" {
          disable-tunnel: [w531 w538] -> w433
          disable-tunnel: [w530 w537] -> w432
          disable-tunnel: w430 -> [w529 w537]
          disable-tunnel: w429 -> [w528 w538]
          frame Disabled {
            w527 = -90.0 ("angle")
            w534 = u16 0 items=["degree", "radians"] ("angle unit")
            n140 = call <vilib>:"Rotate Y-axis.vi"("angle unit"=w534, "Relative?"=FALSE, "error in (no error)"=w529, "angle"=w527, "Scene Object In"=w528) -> ("error out"=w536:errorcluster, "Scene Object Out"=w535:refnum<vi>)  [unwired: 5 in]
            n141 = call <vilib>:"Rotate Z-axis.vi"("angle unit"=w534, "Relative?"=TRUE, "error in (no error)"=w536, "angle"=w527, "Scene Object In"=w535) -> ("error out"=w530:errorcluster, "Scene Object Out"=w531:refnum<vi>)  [unwired: 5 in]
          }
          frame Enabled {
          }
        }
        n142 = call <vilib>:"Create Sphere.vi"("Radius"=sgl 6378.14) -> ("New Sphere Refnum"=w451:refnum<vi>)  [unwired: 9 in, 1 out]
        n143 = call-poly <vilib>:"Add Object.vi"("error in (no error)"=w485, "New Object In"=w488, "Scene Object In"=w487) -> ("error out"=w465:errorcluster, "Scene Object Out"=w466:refnum<vi>)  [unwired: 7 in]
        n144 = invoke class="SceneObject" method="Set Drawable"(reference=w417, error in=w416, "Drawable"=w451) -> (reference out=w449:refnum<vi>, error out=w448:errorcluster)  [unwired: 1 in, 2 out]
        n145 = Bundle By Name(cluster=cluster{"A":sgl, "B":sgl, "C":sgl, "D":sgl} {"A"=0.0, "B"=0.0, "C"=0.0, "D"=0.0} ("Plane"), "A"=w475, "B"=w475, "C"=sgl 1.0 ("B"), "D"=sgl 0.01 ("B")) -> (w472:cluster{"A":sgl, "B":sgl, "C":sgl, "D":sgl})
        n146 = call <vilib>:"Set Translation.vi"("error in (no error)"=w435, "Translation"=cluster{"X":sgl, "Y":sgl, "Z":sgl} {"X"=0.0, "Y"=0.0, "Z"=0.0}, "Scene Object"=w436) -> ("error out"=w438:errorcluster, "Translated Object"=w437:refnum<vi>)  [unwired: 7 out]
        n147 = call <vilib>:"Create Clip Plane.vi"("error in (no error)"=w465, "Number"=0, "Plane"=w472) -> ("error out"=w468:errorcluster, "New Clip Plane Refnum"=w470:refnum<vi>)  [unwired: 7 out]
        n148 = call <vilib>:"Set Translation.vi"("error in (no error)"=w432, "Translation"=cluster{"X":sgl, "Y":sgl, "Z":sgl} {"X"=0.0, "Y"=0.0, "Z"=0.0}, "Scene Object"=w433) -> ("error out"=w428:errorcluster, "Translated Object"=w427:refnum<vi>)  [unwired: 7 out]
        n149 = disable-structure shown="Enabled" {
          disable-tunnel: w449 -> [w520 w524]
          disable-tunnel: w448 -> [w517 w523]
          disable-tunnel: [w516 w522] -> w442
          disable-tunnel: [w515 w521] -> w441
          disable-tunnel: w418 -> [_ w525]
          frame Disabled {
            n150 = property class="SceneObject"(reference=w520, error in=w517, "Draw Style.Line Width"=sgl 2.0 ("Draw Style:Line Width"), "Draw Style.Mode"=T5."Wireframe" ("Draw Style:Mode")) -> (reference out=w516:refnum<vi>, error out=w515:errorcluster)
          }
          frame Enabled {
            n151 = call-poly <vilib>:"Apply Texture.vi"("error in (no error)"=w523, "Apply Mode"=T4."As a replacement", "Image Data"=w525, "Scene Object In"=w524) -> ("error out"=w521:errorcluster, "Scene Object Out"=w522:refnum<vi>)  [unwired: 6 in]
          }
        }
        n152 = Merge Errors(w438, w453) -> (w457:errorcluster)
        n153 = call-poly <vilib>:"Add Object.vi"("error in (no error)"=w457, "New Object In"=w454, "Scene Object In"=w437) -> ("error out"=w455:errorcluster, "Scene Object Out"=w456:refnum<vi>)  [unwired: 7 in]
        n154 = call-poly <vilib>:"Set Clip Plane.vi"("error in (no error)"=w468, "Clip Plane State"=enum16{"Inherit Value", "Off", "On"}."Off", "Clip Plane Refnum In"=w470, "Scene Object In"=w466) -> ("error out"=w445:errorcluster, "Scene Object Out"=w443:refnum<vi>)  [unwired: 6 in]
        n155 = Merge Errors(w445, w441) -> (w447:errorcluster)
        n156 = call-poly <vilib>:"Add Object.vi"("error in (no error)"=w447, "New Object In"=w442, "Scene Object In"=w443) -> ("error out"=w446:errorcluster, "Scene Object Out"=w444:refnum<vi>)  [unwired: 7 in]
        n157 = Merge Errors(w446, w455) -> (w478:errorcluster)
        n158 = call-poly <vilib>:"Add Object.vi"("error in (no error)"=w478, "New Object In"=w456, "Scene Object In"=w444) -> ("error out"=w461:errorcluster, "Scene Object Out"=w464:refnum<vi>)  [unwired: 7 in]
        n159 = Merge Errors(w461, w428) -> (w460:errorcluster)
        n160 = call-poly <vilib>:"Add Object.vi"("error in (no error)"=w460, "New Object In"=w427, "Scene Object In"=w464) -> ("Scene Object Out"=w425:refnum<vi>)  [unwired: 7 in, 1 out]
      }
    }
    "3D Picture Control" <- w2
    n161 = Wait Until Next ms Multiple(millisecond multiple=u32 10) -> ()  [unwired: 1 out]
  }
